vi "Robot_volume_compute.vi"() -> (3 "Volume (m^3)":dbl)   [LabVIEW 2015]
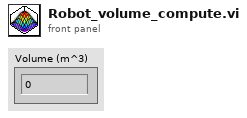
[diagram p1: front panel]
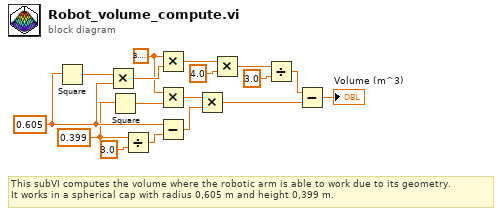
[diagram p0: block diagram]
diagram:
  w5 = 0.399 ("x^2")
  w9 = 3.141592653589793
  w7 = 0.605
  # "This subVI computes the volume where the robotic arm is able to work due to its geometry.\nIt works in a spherical cap with radius 0,605 m and height 0,399 m."
  n1 = Square(x=w7) -> (x^2=w17:dbl)
  n2 = Multiply(x=w17, y=w7) -> (x*y=w16:dbl)
  n3 = Square(x=w5) -> (x^2=w10:dbl)
  n4 = Divide(x=w5, y=3.0) -> (x/y=w4:dbl)
  n5 = Multiply(x=w9, y=w16) -> (x*y=w15:dbl)
  n6 = Multiply(x=w9, y=w10) -> (x*y=w8:dbl)
  n7 = Subtract(x=w7, y=w4) -> (x-y=w3:dbl)
  n8 = Multiply(x=w8, y=w3) -> (x*y=w2:dbl)
  n9 = Multiply(x=w15, y=4.0) -> (x*y=w13:dbl)
  n10 = Divide(x=w13, y=3.0) -> (x/y=w11:dbl)
  n11 = Subtract(x=w11, y=w2) -> (x-y=→"Volume (m^3)":dbl)
